vi "Destination Bounds.vi"() -> (3 "Destination Bounds":T1)   [LabVIEW 2020, in "Better Search.lvlib" / "BetterSearch.lvclass"]
uses:
  BetterSearch.lvclass
  <vilib>/Utility/miscctls.llb/LVRectTypeDef.ctl
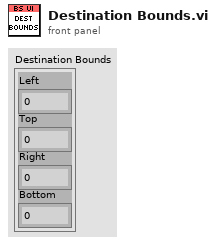
[diagram p1: front panel]
types:
  T1 = typedef "LVRectTypeDef.ctl" = cluster{"Left":i16, "Top":i16, "Right":i16, "Bottom":i16}
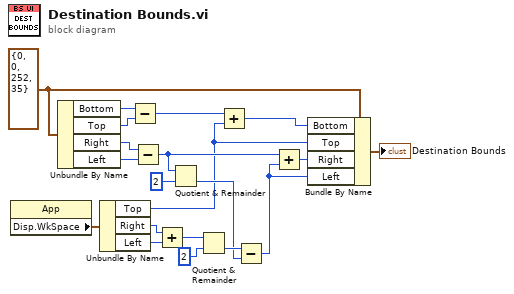
[diagram p0: block diagram]
diagram:
  w11 = T1 {"Left"=0, "Top"=0, "Right"=252, "Bottom"=35} ("Front Panel Window:Panel Bounds")
  n1 = property class="App"() -> ("Disp.WkSpace"=w7:T1)  [unwired: 2 in, 2 out]
  n2 = Unbundle By Name(w11) -> ("Bottom"=w6:i16, "Top"=w5:i16, "Right"=w14:i16, "Left"=w15:i16)
  n3 = Unbundle By Name(w7) -> ("Top"=w3:i16, "Right"=w20:i16, "Left"=w19:i16)
  n4 = Subtract(x=w6, y=w5) -> (x-y=w4:i16)
  n5 = Subtract(x=w14, y=w15) -> (x-y=w9:i16)
  n6 = Add(x=w20, y=w19) -> (x+y=w18:i16)
  n7 = Quotient & Remainder(x=w9, y=i16 2) -> (floor(x/y)=w12:i16)  [unwired: 1 out]
  n8 = Quotient & Remainder(x=w18, y=i16 2) -> (floor(x/y)=w13:i16)  [unwired: 1 out]
  n9 = Add(x=w4, y=w3) -> (x+y=w2:i16)
  n10 = Subtract(x=w13, y=w12) -> (x-y=w10:i16)
  n11 = Add(x=w9, y=w10) -> (x+y=w8:i16)
  n12 = Bundle By Name(cluster=w11, "Bottom"=w2, "Top"=w3, "Right"=w8, "Left"=w10) -> (→"Destination Bounds":T1)
